vi "XNETInterfaceDiscover.vi"() -> (2 "CAN":cluster{"Interface":refnum<k21>[], "Slot":u32[]})   [LabVIEW 2021]
uses:
  <resource>/objmgr/xnet.rc
panel:
  in  "error in":errorcluster
  out "error out":errorcluster
  out "iteration":i32
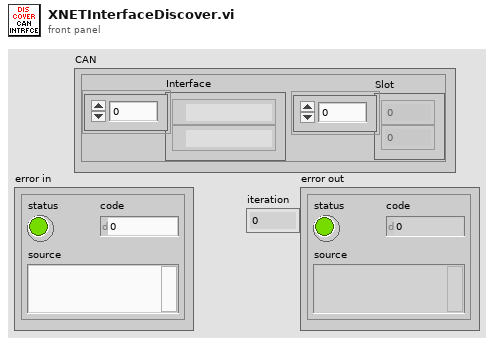
[diagram p1: front panel]
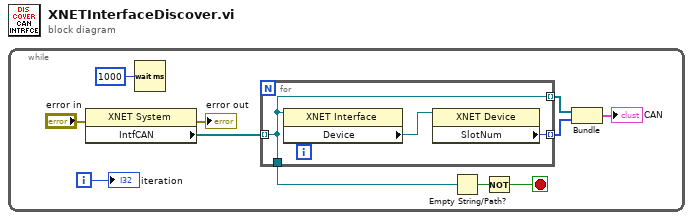
[diagram p0: block diagram]
diagram:
  n1 = while {
    i -> [w8]
    stop <- w6 stop-if-true
    n2 = property class="XNET System"(error in="error in") -> (error out=→"error out":errorcluster, "IntfCAN"=w11:refnum<k21>[])  [unwired: 1 in, 1 out]
    n3 = Wait (ms)(milliseconds to wait=u32 1000) -> ()  [unwired: 1 out]
    n4 = for {
      tunnel: w11 -> [w12] mode=indexing
      tunnel: [w12] -> w5 mode=indexing
      tunnel: [w13] -> w4 mode=indexing
      tunnel: [w12] -> w7
      n5 = property class="XNET Interface"(reference=w12) -> ("Device"=w14:refnum<k21>)  [unwired: 1 in, 2 out]
      n6 = property class="XNET Device"(reference=w14) -> ("SlotNum"=w13:u32)  [unwired: 1 in, 2 out]
    }
    n7 = Empty String/Path?(string/path=w7) -> (empty?=w9:bool)
    n8 = Not(x=w9) -> (.not. x?=w6:bool)
    n9 = Bundle(w5, w4) -> (→"CAN":cluster{refnum<k21>[], u32[]})  [unwired: 1 in]
    "iteration" <- w8
  }
